vi "walk out.vi"(0 "Number of sets of steps":i32=6, 1 "Walk out number steps":u16=10, 2 "Walk out Amplitude (V)":sgl=320.0) -> ()   [LabVIEW 2021]
uses:
  <userlib>/Nanonis Prog Interface V5/Nanonis Prog Interface.lvlib
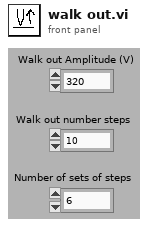
[diagram p1: front panel]
types:
  T1 = enum8{"Group 1", "Group 2", "Group 3", "Group 4", "Group 5", "Group 6"}
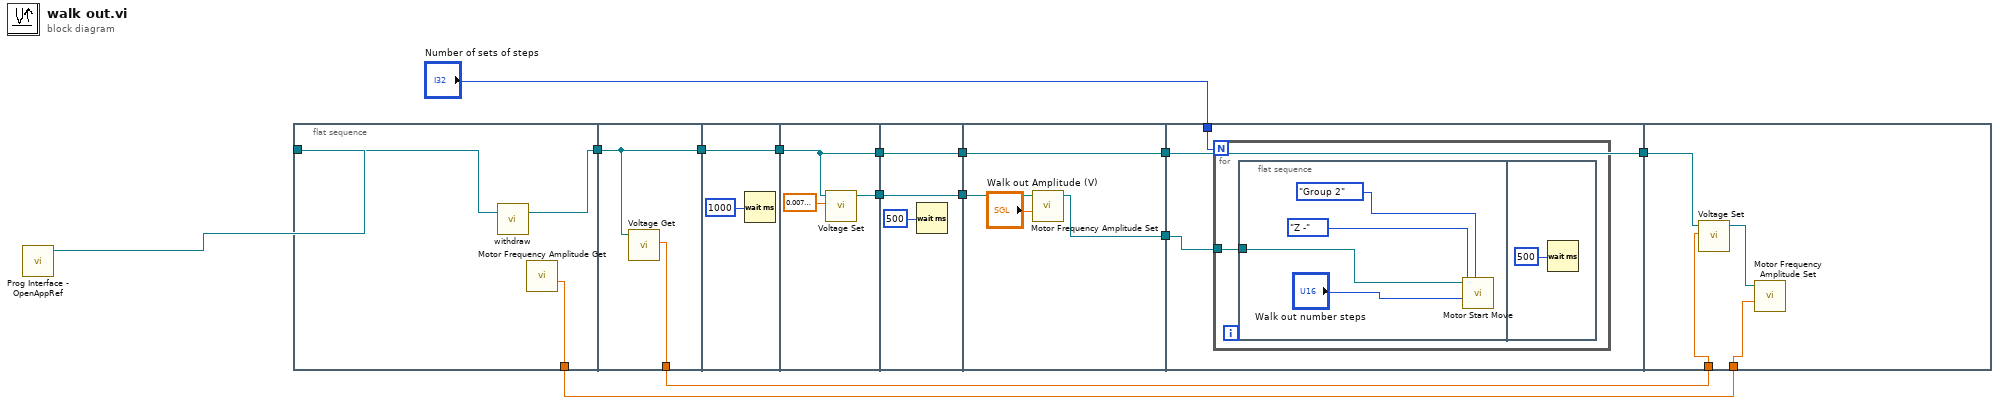
[diagram p0: block diagram]
diagram:
  n1 = call <userlib>:"Prog Interface - OpenAppRef.vi"() -> ("Application reference"=w14:refnum<vi>)  [unwired: 6 in, 1 out]
  n2 = flat-sequence {
    tunnel: [w15] -> w13
    tunnel: [w17] -> w1
    tunnel: w14 -> [w16]
    tunnel: w13 -> [w19]
    tunnel: [w19] -> w12
    tunnel: [w18] -> w2
    tunnel: w12 -> [w21]
    tunnel: [w21] -> w11
    tunnel: [w23] -> w10
    tunnel: w11 -> [w22]
    tunnel: [w22] -> w9
    tunnel: w10 -> [w27]
    tunnel: [w27] -> w8
    tunnel: [w25] -> w7
    tunnel: w9 -> [w25]
    tunnel: w8 -> [w31]
    tunnel: [w30] -> w6
    tunnel: [w28] -> w5
    tunnel: w7 -> [w28]
    tunnel: w6 -> [w34]
    tunnel: "Number of sets of steps" -> [w33]
    tunnel: [w32] -> w4
    tunnel: w5 -> [w32]
    tunnel: w1 -> [w42]
    tunnel: w2 -> [w43]
    tunnel: w4 -> [w44]
    frame #0 {
      n3 = call "withdraw.vi"("Application ref in"=w16) -> ("Application ref out"=w15:refnum<vi>)  [unwired: 2 in]
      n4 = call <userlib>:"Motor Frequency Amplitude Get.vi"() -> ("Amplitude (V)"=w17:sgl)  [unwired: 8 in, 3 out]
    }
    frame #1 {
      n5 = call <userlib>:"Voltage Get.vi"("Application ref in"=w19) -> ("Bias (V)"=w18:sgl)  [unwired: 8 in, 2 out]
    }
    frame #2 {
      n6 = Wait (ms)(milliseconds to wait=u32 1000) -> ()  [unwired: 1 out]
    }
    frame #3 {
      n7 = call <userlib>:"Voltage Set.vi"("Bias (V)"=sgl 0.007, "Application ref in"=w22) -> ("Application ref out"=w23:refnum<vi>)  [unwired: 8 in, 1 out]
    }
    frame #4 {
      n8 = Wait (ms)(milliseconds to wait=u32 500) -> ()  [unwired: 1 out]
    }
    frame #5 {
      n9 = call <userlib>:"Motor Frequency Amplitude Set.vi"("Amplitude (V) (NaN=no change)"="Walk out Amplitude (V)", "Application ref in"=w31) -> ("Application ref out"=w30:refnum<vi>)  [unwired: 8 in, 1 out]
    }
    frame #6 {
      n10 = for {
        N: w33 -> [_]
        tunnel: w34 -> [w35]
        n11 = flat-sequence {
          tunnel: w35 -> [w37]
          frame #0 {
            n12 = call <userlib>:"Motor Start Move.vi"("Group"=T1."Group 2", "Number of steps"="Walk out number steps", "Direction"=enum16{"X +", "X -", "Y +", "Y -", "Z +", "Z -"}."Z -", "Application ref in"=w37) -> ()  [unwired: 5 in, 2 out]
          }
          frame #1 {
            n13 = Wait (ms)(milliseconds to wait=u32 500) -> ()  [unwired: 1 out]
          }
        }
      }
    }
    frame #7 {
      n14 = call <userlib>:"Voltage Set.vi"("Bias (V)"=w43, "Application ref in"=w44) -> ("Application ref out"=w41:refnum<vi>)  [unwired: 8 in, 1 out]
      n15 = call <userlib>:"Motor Frequency Amplitude Set.vi"("Amplitude (V) (NaN=no change)"=w42, "Application ref in"=w41) -> ()  [unwired: 8 in, 2 out]
    }
  }
